vi "Add Step To End.vi"(6 "Step Name":string, 7 "Reply Channel":refnum<notifier>, 8 "error in (no error)":errorcluster, 10 "Parameter":variant, 11 "Actor in":refnum<class "Actor.lvclass">) -> (0 "error out":errorcluster, 3 "Actor out":refnum<class "Actor.lvclass">)   [LabVIEW 2015, in "Actor.lvclass"]
uses:
  Actor.lvclass
  Messaging/Message/Message.lvclass
  Actor.lvclass/Actor.ctl
  Sequencer/Sequencer.lvclass
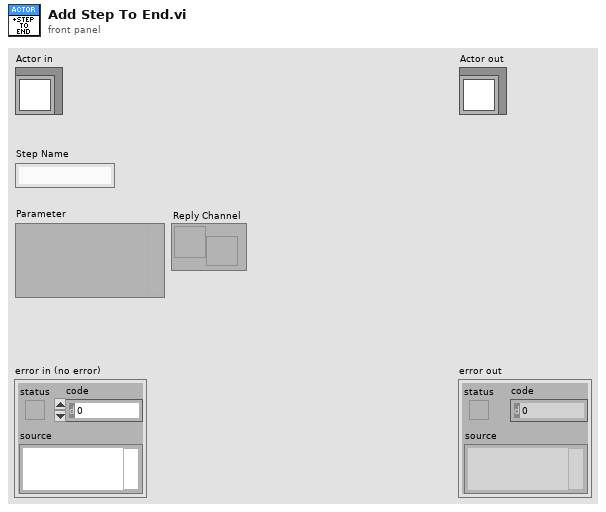
[diagram p1: front panel]
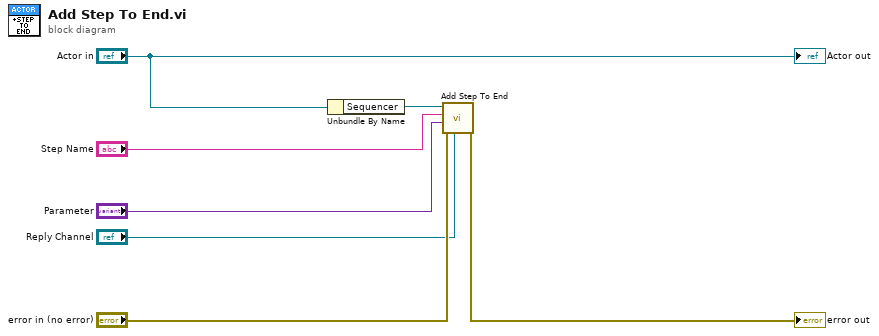
[diagram p0: block diagram]
diagram:
  n1 = Unbundle By Name("Actor in") -> ("Sequencer"=w1:refnum<class "Sequencer.lvclass">)
  n2 = call "Add Step To End.vi"("Reply Channel"="Reply Channel", "error in (no error)"="error in (no error)", "Parameter"="Parameter", "Step Name"="Step Name", "Sequencer in"=w1) -> ("error out"=→"error out":errorcluster)  [unwired: 6 in]
  "Actor out" <- "Actor in"
